vi "Periodic Tasks.vi"(8 "error in":errorcluster) -> ()   [LabVIEW 2017]
doc: "This VI runs in parallel to other tasks. It can contain as many user-defined periodic loops as you need. These can carry out PID or other sorts of timed response."
uses:
  Public/Documents/Cross The Road Electronics/Phoenix-LabVIEW/Motor Controller/Controls/CTRE_Phoenix_MotorControl_ControlMode.ctl
  Robot Global Data.vi
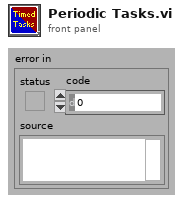
[diagram p1: front panel]
types:
  T1 = typedef "CTRE_Phoenix_MotorControl_ControlMode.ctl" = u16
  T2 = typedef "WPI_JoystickDevRef.ctl" = cluster{"Device":T3}
  T3 = typedef "WPI_JoystickDeviceEnum.ctl" = enum16{"USB 0", "USB 1", "USB 2", "USB 3", "USB 4", "USB 5"}
  T4 = typedef "WPI_RobotDriveDevRef.ctl" = cluster{"DevStatus":errorcluster, "Motors[]":T5[], "Square Inputs":bool, "Max Output":dbl}
  T5 = typedef "WPI_MotorControlDeviceRef.ctl" = cluster{"DeviceStatus":errorcluster, "Type":T6, "PWM":cluster{"PWM Channel":T7, "DeadBand":T8}, "CAN":cluster{"Device Number":u8, "SetOutput VI Ref":variant, "GetOutput VI Ref":variant, "Enable VI Ref":variant, "Disable VI Ref":variant, "Data":variant}, "Invert":bool, "DIO PWM":cluster{"PWM \"Enable\" Channel":T7, "DIOChannel":T9, "PWM Rate":dbl}}
  T6 = typedef "WPI_MotorControlType.ctl" = enum16{"PWM", "CAN", "DIO PWM"}
  T7 = typedef "FPGA_DIOPWMChannel.ctl" = enum8{"PWM 0", "PWM 1", "PWM 2", "PWM 3", "PWM 4", "PWM 5", "PWM 6", "PWM 7", "PWM 8", "PWM 9", "PWM MXP 0", "PWM MXP 1", "PWM MXP 2", "PWM MXP 3", "PWM MXP 4", "PWM MXP 5", "PWM MXP 6", "PWM MXP 7", "PWM MXP 8", "PWM MXP 9", "Invalid"}
  T8 = typedef "WPI_PWMDeadband.ctl" = cluster{"Name":string, "maxPositivePwm":i32, "minPositivePwm":i32, "centerPwm":i32, "maxNegativePwm":i32, "minNegativePwm":i32, "angularRange":u16}
  T9 = typedef "FPGA_DIOChannel.ctl" = enum8{"DIO 0", "DIO 1", "DIO 2", "DIO 3", "DIO 4", "DIO 5", "DIO 6", "DIO 7", "DIO 8", "DIO 9", "DIO MXP 0", "DIO MXP 1", "DIO MXP 2", "DIO MXP 3", "DIO MXP 4", "DIO MXP 5", "DIO MXP 6", "DIO MXP 7", "DIO MXP 8", "DIO MXP 9", "DIO MXP 10", "DIO MXP 11", "DIO MXP 12", "DIO MXP 13", "DIO MXP 14", "DIO MXP 15", "SPI Port CS1", "SPI Port CS2", "SPI Port CS3", "SPI Port MISO", "SPI Port MOSI", "Invalid"}
  T10 = cluster{"JoystickDevRef":T2, "RobotDriveDevRef":T4}
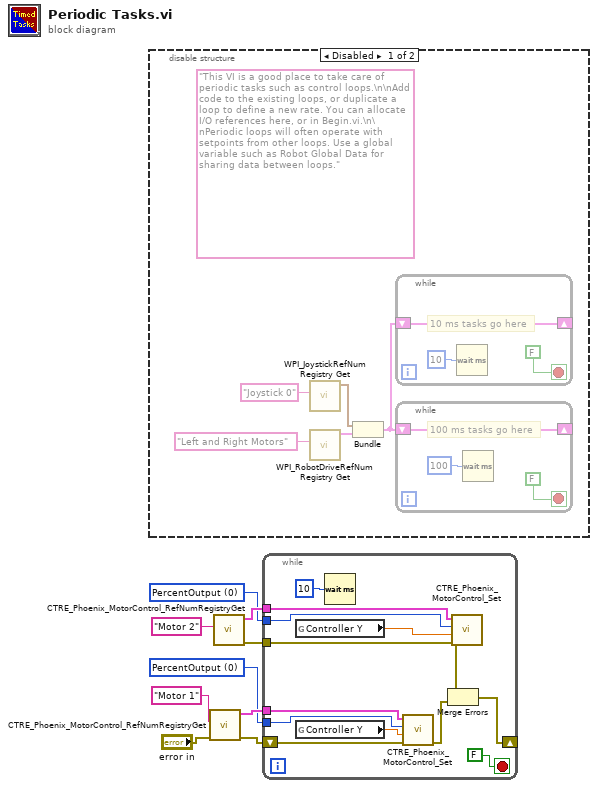
[diagram p0: block diagram]
diagram:
  w2 = T1 0 items=["PercentOutput"=0, "Position"=1, "Velocity"=2, "Current"=3, "Follower"=5, "MotionProfile"=6, "MotionMagic"=7, "MotionMagicArc"=8, "MotionProfileArc"=10, "Disabled"=15] ("Control Mode")
  w6 = T1 0 items=["PercentOutput"=0, "Position"=1, "Velocity"=2, "Current"=3, "Follower"=5, "MotionProfile"=6, "MotionMagic"=7, "MotionMagicArc"=8, "MotionProfileArc"=10, "Disabled"=15] ("Control Mode")
  n1 = disable-structure shown="Disabled" {
    frame Disabled {
      (unwired) "This VI is a good place to take care of periodic tasks such as control loops.\n\nAdd code to the existing loops, or duplicate a loop to define a new rate. You can allocate I/O references here, or in Begin.vi.\n\nPeriodic loops will often operate with setpoints from other loops. Use a global variable such as Robot Global Data for sharing data between loops."
      n2 = call <vilib>:"WPI_JoystickRefNum Registry Get.vi"("refnum name"="Joystick 0") -> ("JoystickDevRef"=w12:T2)  [unwired: 1 in, 9 out]
      n3 = call <vilib>:"WPI_RobotDriveRefNum Registry Get.vi"("refnum name"="Left and Right Motors") -> ("RobotDriveDevRef"=w11:T4)  [unwired: 1 in, 9 out]
      n4 = Bundle("JoystickDevRef"=w12, "RobotDriveDevRef"=w11) -> (w10:T10)  [unwired: 1 out]
      n5 = while {
        shift-right: [w18] -> _
        shift-left: w10 -> [w18]
        stop <- FALSE stop-if-true
        # "10 ms tasks go here"
        n6 = Wait (ms)(milliseconds to wait=u32 10) -> ()  [unwired: 1 out]
      }
      n7 = while {
        shift-right: [w15] -> _
        shift-left: w10 -> [w15]
        stop <- FALSE stop-if-true
        # "100 ms tasks go here"
        n8 = Wait (ms)(milliseconds to wait=u32 100) -> ()  [unwired: 1 out]
      }
    }
    frame Enabled {
    }
  }
  n9 = call "CTRE_Phoenix_MotorControl_RefNumRegistryGet.vi"("error in (no error)"="error in", "refnum name"="Motor 1") -> ("error out"=w7:errorcluster, "PhoenixMotorControlDevRef"=w9:T5)  [unwired: 8 in]
  n10 = call "CTRE_Phoenix_MotorControl_RefNumRegistryGet.vi"("refnum name"="Motor 2") -> ("error out"=w3:errorcluster, "PhoenixMotorControlDevRef"=w4:T5)  [unwired: 9 in]
  n11 = while {
    tunnel: w9 -> [w33]
    tunnel: w6 -> [w31]
    tunnel: w4 -> [w30]
    tunnel: w3 -> [w29]
    tunnel: w2 -> [w28]
    shift-right: [w22] -> _
    shift-left: w7 -> [w32]
    stop <- FALSE stop-if-true
    n12 = global read "Robot Global Data.vi" "Controller Y"() -> (w21:dbl)
    n13 = global read "Robot Global Data.vi" "Controller Y"() -> (w27:dbl)
    n14 = Wait (ms)(milliseconds to wait=10) -> ()  [unwired: 1 out]
    n15 = call "CTRE_Phoenix_MotorControl_Set.vi"("error in (no error)"=w32, "Output"=w27, "Control Mode"=w31, "PhoenixMotorControlDevRef"=w33) -> ("error out"=w23:errorcluster)  [unwired: 6 in, 1 out]
    n16 = call "CTRE_Phoenix_MotorControl_Set.vi"("error in (no error)"=w29, "Output"=w21, "Control Mode"=w28, "PhoenixMotorControlDevRef"=w30) -> ("error out"=w24:errorcluster)  [unwired: 6 in, 1 out]
    n17 = Merge Errors(w24, w23) -> (w22:errorcluster)
  }
